vi "Modulation.vi"() -> ()   [LabVIEW 2017]
uses:
  <vilib>/sound2/lvsound2.llb/Sound Data Format.ctl
  <vilib>/sound2/lvsound2.llb/Sampling Mode.ctl
  <vilib>/Utility/error.llb/DialogType.ctl
  <vilib>/express/express analysis/Spectral/Block/exnSpectralBlock spectral measurements power poly.vi
  <vilib>/express/express analysis/Spectral/Block/exnSpectralBlock spectral measurements power WFM.vi
  <vilib>/sound2/lvsound2.llb/Sound Output Write (DBL Single).vi
  <vilib>/express/express analysis/Spectral/XNode/ExpressSpectralMeasurementsBlockNode.xnode
  <vilib>/Analysis/NI_AALPro.lvlib
panel:
  in  "Modulationsart":enum16{"AM", "FM", "PM"}(ring)
  in  "Stop":bool
  out "Waveform Graph 2":cluster{"f0":dbl, "df":dbl, "magnitude":dbl[]}(graph)={"f0"=0.0, "df"=1.0, "magnitude"=array[5000 elements]}
  out "Waveform Graph":waveform(dbl)(graph)
  in  "Modulationsgrad m (k)":dbl=1.0
  in  "Amplitude 2 (Mod.)":dbl
  in  "Frequenz 2 (Mod.)":dbl
  in  "Amplitude 1 (Mod.)":dbl=1.0
  in  "Frequenz 1 (Mod.)":dbl=5.0
  in  "Frequenz (Träger)":dbl=50.0
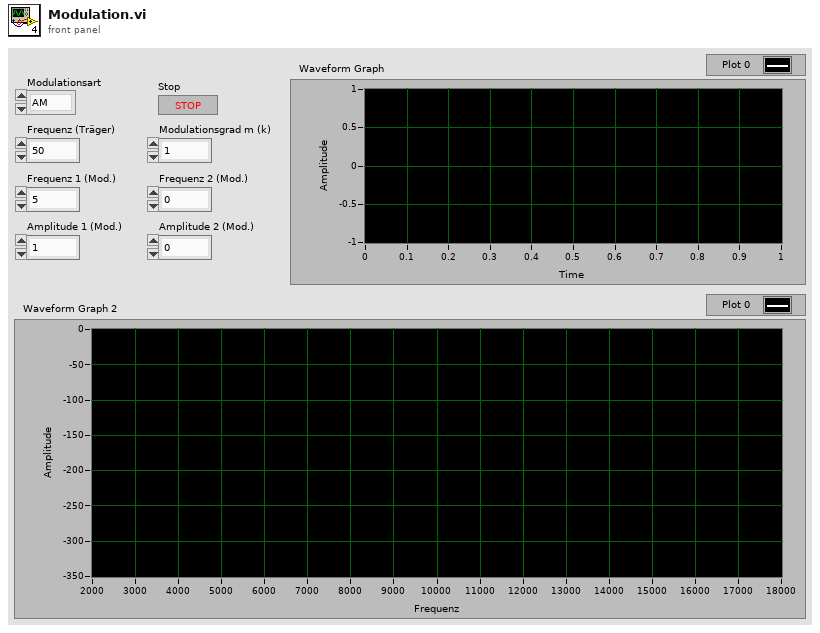
[diagram p1: front panel]
types:
  T1 = typedef "Sampling Mode.ctl" = i32
  T2 = typedef "Sound Data Format.ctl" = cluster{"sample rate (S/s)":dbl, "number of channels":i32, "bits per sample":i32}
  T3 = typedef "Sound Output Task ID.ctl" = u32
  T4 = cluster{"averaging mode":u16, "weighting mode":u16, "number of averages":u32}
  T5 = cluster{"dB On (F)":bool, "unwrap phase (F)":bool, "convert to degree (F)":bool}
  T6 = typedef "DialogType.ctl" = u16
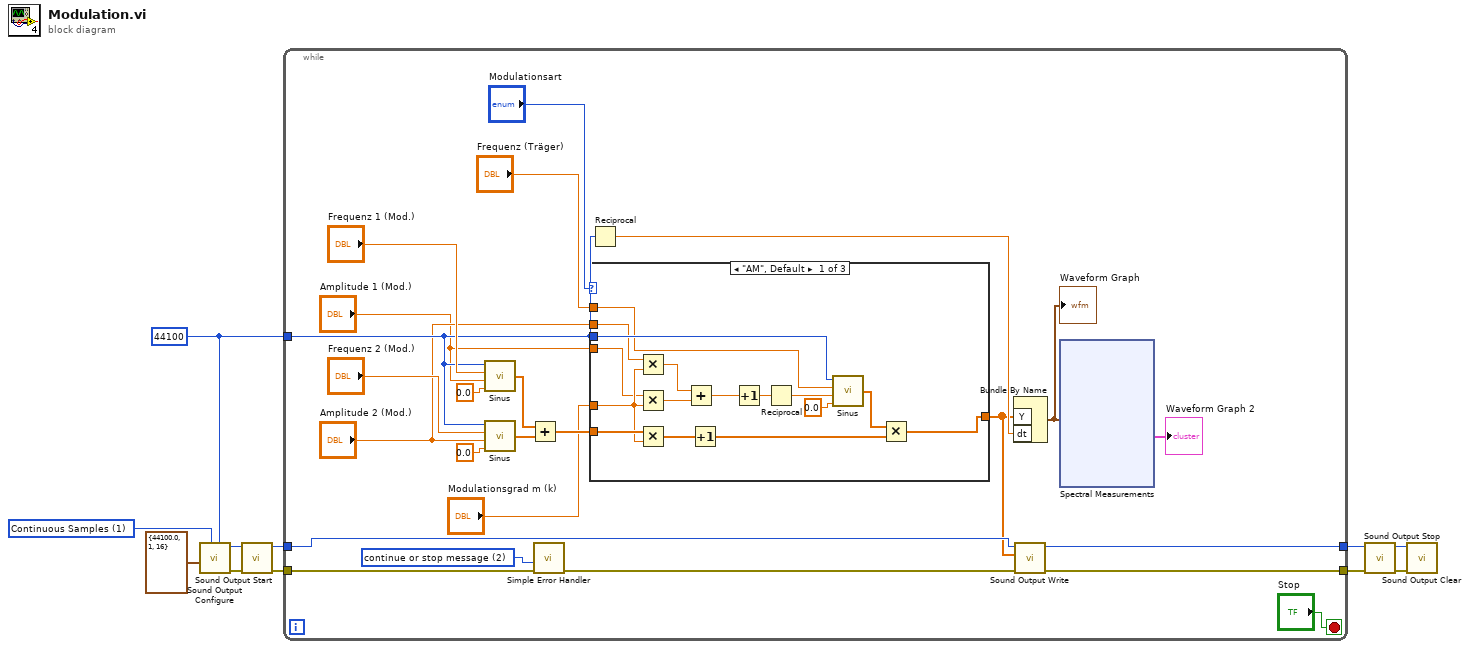
[diagram p0: block diagram]
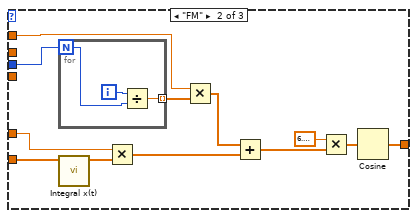
[diagram p2: hidden frame]
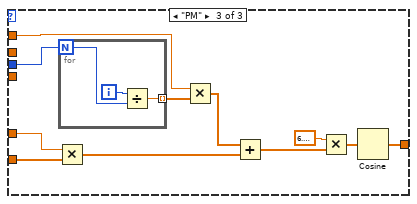
[diagram p3: hidden frame]
diagram:
  w1 = 44100 ("number of samples/ch")
  w5 = T1 1 items=["Finite Samples", "Continuous Samples"] ("sample mode")
  n1 = call <vilib>:"Sound Output Configure.vi"("number of samples/ch"=w1, "sample mode"=w5, "sound format"=T2 {"sample rate (S/s)"=44100.0, "number of channels"=1, "bits per sample"=16}) -> ("error out"=w6:errorcluster, "task ID"=w7:T3)  [unwired: 7 in]
  n2 = call <vilib>:"Sound Output Start.vi"("error in (no error)"=w6, "task ID"=w7) -> ("error out"=w3:errorcluster, "task ID out"=w2:T3)  [unwired: 8 in]
  n3 = while {
    tunnel: [w24] -> w10
    tunnel: [w23] -> w9
    tunnel: w3 -> [w20]
    tunnel: w2 -> [w19]
    tunnel: w1 -> [w18]
    stop <- "Stop" stop-if-true
    w27 = T6 2 items=["no dialog", "OK message", "continue or stop message", "OK message + warnings", "continue/stop + warnings"] ("type of dialog (OK msg:1)")
    n4 = call "Sinus.vi"("Phase phi"=0.0 ("Phase (Mod.)"), "Amplitude A"="Amplitude 1 (Mod.)", "Frequenz f"="Frequenz 1 (Mod.)", "Datenpunkte N"=w18) -> ("sin(t_i)"=w32:dbl[])
    n5 = call "Sinus.vi"("Phase phi"=0.0 ("Phase (Mod.)"), "Amplitude A"="Amplitude 2 (Mod.)", "Frequenz f"="Frequenz 2 (Mod.)", "Datenpunkte N"=w18) -> ("sin(t_i)"=w33:dbl[])
    n6 = Add(x=w32, y=w33) -> (x+y=w31:dbl[])
    n7 = call <vilib>:"Simple Error Handler.vi"("type of dialog (OK msg:1)"=w27, "error in (no error)"=w20) -> ("error out"=w28:errorcluster)  [unwired: 3 in, 4 out]
    n8 = Reciprocal(x=w18) -> (1/x=w26:dbl)
    n9 = case shown="\"AM\", Default" "Modulationsart" {
      tunnel: w31 -> [w50 w53 w74]
      tunnel: w18 -> [w46 w55 w77]
      tunnel: "Modulationsgrad m (k)" -> [w45 w56 w67]
      tunnel: "Amplitude 1 (Mod.)" -> [w44 _ _]
      tunnel: "Amplitude 2 (Mod.)" -> [w43 _ _]
      tunnel: [w37 w54 w68] -> w16
      tunnel: "Frequenz (Träger)" -> [w36 w57 w75]
      frame "AM", Default {
        n10 = Multiply(x=w43, y=w45) -> (x*y=w41:dbl)
        n11 = Multiply(x=w44, y=w45) -> (x*y=w42:dbl)
        n12 = Multiply(x=w50, y=w45) -> (x*y=w49:dbl[])
        n13 = Add(x=w41, y=w42) -> (x+y=w40:dbl)
        n14 = Increment(x=w49) -> (x+1=w48:dbl[])
        n15 = Increment(x=w40) -> (x+1=w39:dbl)
        n16 = Reciprocal(x=w39) -> (1/x=w38:dbl)
        n17 = call "Sinus.vi"("Phase phi"=0.0 ("Phase (Träger)"), "Amplitude A"=w38, "Frequenz f"=w36, "Datenpunkte N"=w46) -> ("sin(t_i)"=w47:dbl[])
        n18 = Multiply(x=w47, y=w48) -> (x*y=w37:dbl[])
      }
      frame "FM" {
        n19 = for {
          N: w55 -> [w64]
          tunnel: [w65] -> w63 mode=indexing
          i -> [w66]
          n20 = Divide(x=w66, y=w64) -> (x/y=w65:dbl)
        }
        n21 = call <vilib>:"Integral x(t).vi"("X"=w53) -> ("Integral X"=w52:dbl[])  [unwired: 9 in, 1 out]
        n22 = Multiply(x=w56, y=w52) -> (x*y=w62:dbl[])
        n23 = Multiply(x=w57, y=w63) -> (x*y=w61:dbl[])
        n24 = Add(x=w61, y=w62) -> (x+y=w59:dbl[])
        n25 = Multiply(x=6.283185307179586, y=w59) -> (x*y=w58:dbl[])
        n26 = Cosine(x=w58) -> (cos(x)=w54:dbl[])
      }
      frame "PM" {
        n27 = Multiply(x=w67, y=w74) -> (x*y=w73:dbl[])
        n28 = for {
          N: w77 -> [w78]
          tunnel: [w79] -> w76 mode=indexing
          i -> [w80]
          n29 = Divide(x=w80, y=w78) -> (x/y=w79:dbl)
        }
        n30 = Multiply(x=w75, y=w76) -> (x*y=w72:dbl[])
        n31 = Add(x=w72, y=w73) -> (x+y=w70:dbl[])
        n32 = Multiply(x=6.283185307179586, y=w70) -> (x*y=w69:dbl[])
        n33 = Cosine(x=w69) -> (cos(x)=w68:dbl[])
      }
    }
    n34 = Bundle By Name("Y"=w16, "dt"=w26) -> (w25:waveform(dbl))  [unwired: 1 in]
    "Waveform Graph" <- w25
    n35 = call-poly <vilib>:"Sound Output Write.vi"("error in (no error)"=w28, "data"=w16, "task ID"=w19) -> ("error out"=w24:errorcluster, "task ID out"=w23:T3)  [unwired: 7 in]
    n36 = xnode "Spectral Measurements"("Signals"=w25) -> ("Power Spectrum"=→"Waveform Graph 2":cluster{"f0":dbl, "df":dbl, "magnitude":dbl[]})  [unwired: 1 in, 1 out]
  }
  n37 = call <vilib>:"Sound Output Stop.vi"("error in (no error)"=w10, "task ID"=w9) -> ("error out"=w11:errorcluster, "task ID out"=w8:T3)  [unwired: 8 in]
  n38 = call <vilib>:"Sound Output Clear.vi"("error in (no error)"=w11, "task ID"=w8) -> ()  [unwired: 9 in, 1 out]
